vi "Publish and Subscribe Event-based.vi"() -> ()   [LabVIEW 2020]
uses:
  <userlib>/lvwamp/WAMP Client/WAMP Client.lvclass/WAMP Client.ctl
  <userlib>/lvwamp/WAMP Client/Accessors/Read Daemon Stopped.vi
  <userlib>/lvwamp/WAMP Client/New WebSocket Client.vi
  <userlib>/lvwamp/WAMP Client/WAMP Client.lvclass
panel:
  out "Error URI":string
  out "Callee Error?":bool
  out "Call Result ArgumentKw":string
  out "Call Result Arguments":string[](array[string])
  in  "Call Arguments":string[](array[string])
  in  "Call URI":string="test.topic"
  in  "Call":bool caption="Publish Topic"
  in  "Unsubscribe":bool caption="Publish Topic"
  out "Topic:":string
  out "ArgumentKw Payload":string
  out "Arguments Payload":string[](array[string])
  out "Event received on:":string
  in  "Publish Argument Payload":string[](array[string])
  in  "Subscription URI":string="test.topic"
  in  "Subscribe":bool caption="Publish Topic"
  in  "Disconnect":bool caption="Publish Topic"
  in  "Realm":string="default_realm"
  in  "Topic URI":string="test.topic"
  in  "Publish":bool caption="Publish Topic"
  in  "Port":u16=55555
  in  "Router Address":string="localhost"
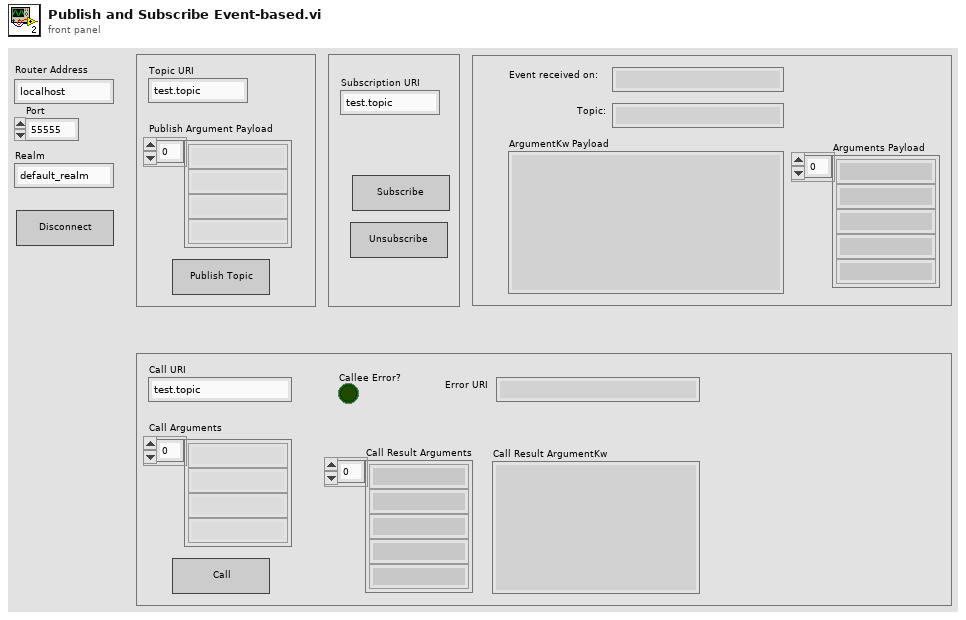
[diagram p1: front panel]
types:
  T1 = typedef "WAMP Client.lvclass/WAMP Error Payload.ctl" = cluster{"Arguments Payload":string[], "ArgumentKw Payload":string, "Error URI":string, "Error?":bool}
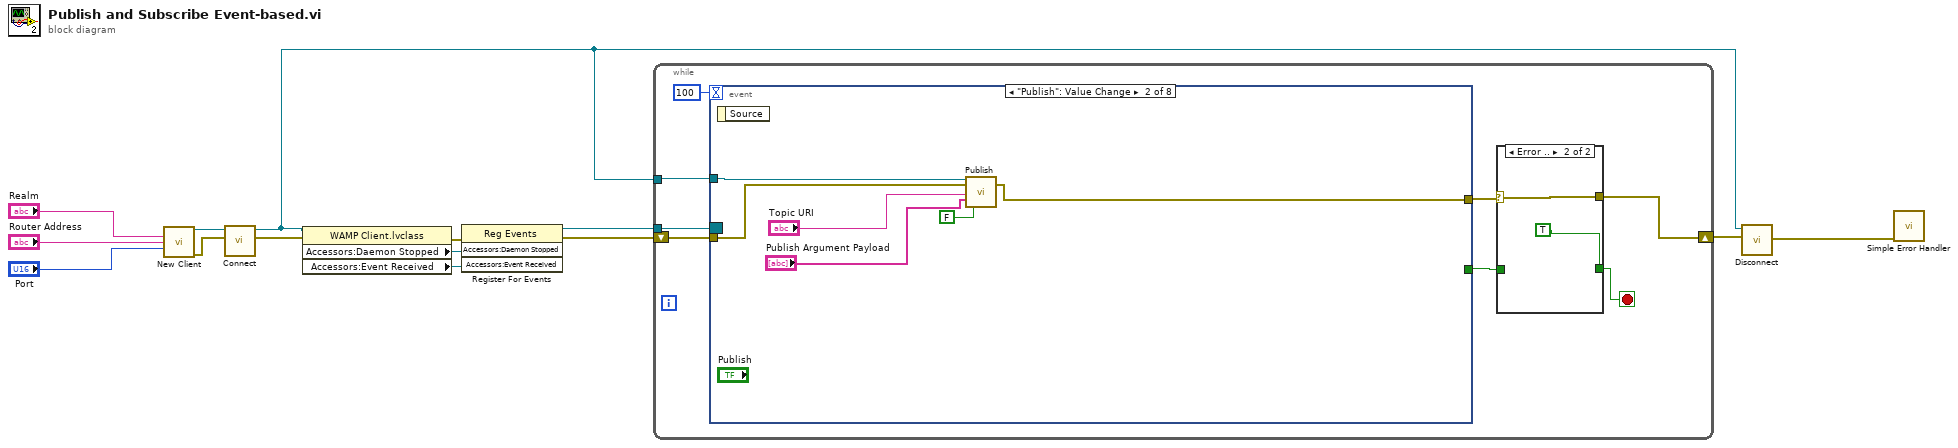
[diagram p0: block diagram]
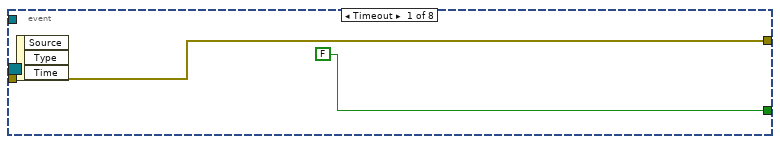
[diagram p3: hidden frame]
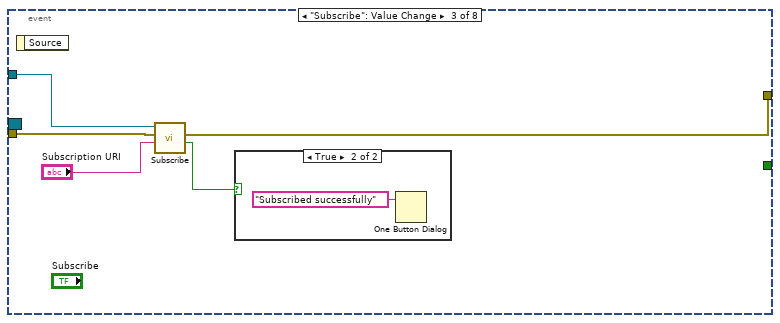
[diagram p4: hidden frame]
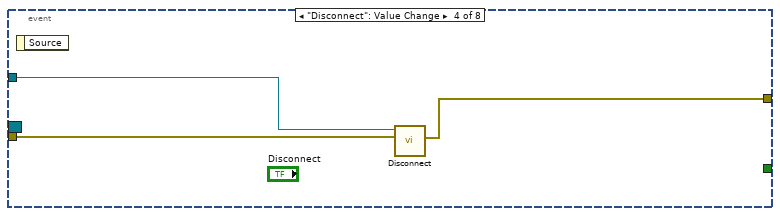
[diagram p6: hidden frame]
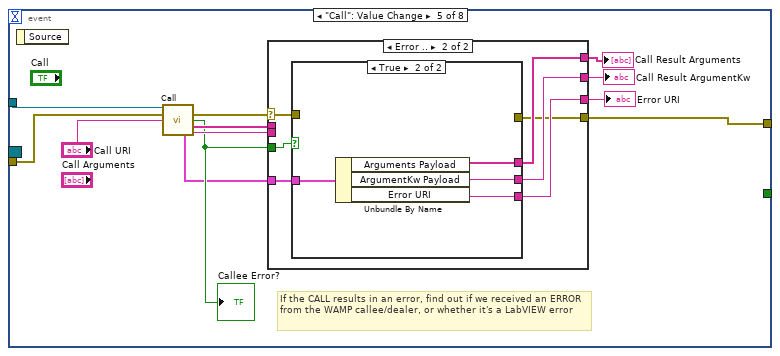
[diagram p7: hidden frame]
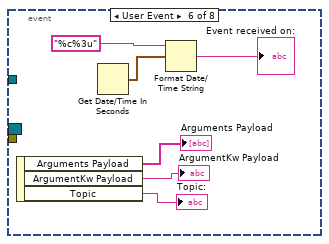
[diagram p10: hidden frame]
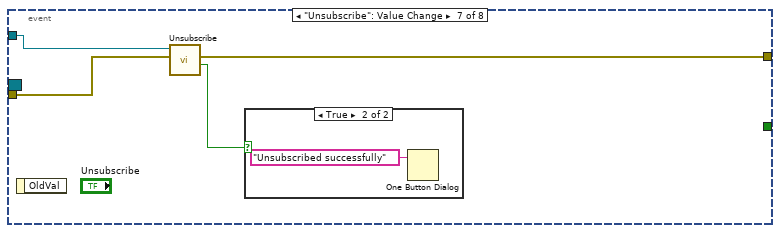
[diagram p11: hidden frame]
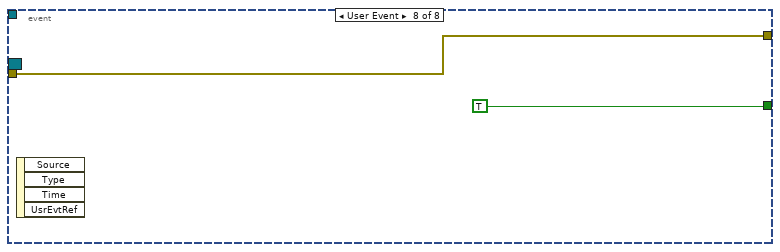
[diagram p13: hidden frame]
diagram:
  n1 = call-poly <userlib>:"New Client.vi"("Realm"="Realm", "Address"="Router Address", "Port"="Port") -> ("reference out"=w11:refnum<class "WAMP Client.lvclass">, "error out"=w8:errorcluster)  [unwired: 11 in]
  n2 = call <userlib>:"Connect.vi"("error in (no error)"=w8, "WAMP Client in"=w11) -> ("error out"=w2:errorcluster, "WAMP Client out"=w3:refnum<class "WAMP Client.lvclass">)  [unwired: 8 in]
  n3 = property class="WAMP Client.lvclass"(reference=w3, error in=w2) -> (error out=w9:errorcluster, "Accessors:Daemon Stopped"=w10:refnum<user-event>, "Accessors:Event Received"=w5:refnum<user-event>)  [unwired: 1 out]
  n4 = register-events(error in=w9, w10, w5) -> (reference out=w6:refnum<event-registration>, error out=w4:errorcluster)  [unwired: 1 in]
  n5 = while {
    tunnel: w3 -> [w22]
    shift-right: [w20] -> w7
    shift-left: w4 -> [w18]
    tunnel: w6 -> [w19]
    stop <- w16 stop-if-true
    n6 = event shown="[1] \"Publish\": Value Change" {
      selector: w19 -> [_ _ _ _ _ _ _ _]
      dyn-events: _ -> [_ _ _ _ _ _ _ _]
      timeout: 100 -> [_ _ _ _ _ _ _ _]
      tunnel: w22 -> [_ w34 w39 w43 w55 _ w79 _]
      tunnel: [FALSE _ _ _ _ _ _ TRUE] -> w17
      tunnel: w18 -> [w27 w33 w38 w41 w54 _ w80 w82]
      tunnel: [w27 w32 w37 w42 w51 _ w78 w82] -> w21
      event Timeout {
        n7 = event-data() -> ()  [unwired: 1 in, 3 out]
      }
      event "Publish": Value Change {
        n8 = event-data() -> ()  [unwired: 1 in, 1 out]
        n9 = call-dynamic "Publish.vi"("WAMP Client in"=w34, "error in (no error)"=w33, "Topic"="Topic URI", "Arguments"="Publish Argument Payload", "Request Ack."=FALSE) -> ("error out"=w32:errorcluster)  [unwired: 13 in, 1 out]
      }
      event "Subscribe": Value Change {
        n10 = event-data() -> ()  [unwired: 1 in, 1 out]
        n11 = call-dynamic "Subscribe.vi"("Topic"="Subscription URI", "error in (no error)"=w38, "WAMP Client in"=w39) -> ("Success?"=w36:bool, "error out"=w37:errorcluster)  [unwired: 3 in, 2 out]
        n12 = case shown="True" w36 {
          frame False {
          }
          frame True {
            n13 = One Button Dialog(message="Subscribed successfully") -> ()  [unwired: 1 in, 1 out]
          }
        }
      }
      event "Disconnect": Value Change {
        n14 = event-data() -> ()  [unwired: 1 in, 1 out]
        n15 = call-dynamic "Disconnect.vi"("error in (no error)"=w41, "WAMP Client in"=w43) -> ("error out"=w42:errorcluster)  [unwired: 8 in, 1 out]
      }
      event "Call": Value Change {
        # "If the CALL results in an error, find out if we received an ERROR from the WAMP callee/dealer, or whether it's a LabVIEW error"
        n16 = event-data() -> ()  [unwired: 1 in, 1 out]
        n17 = call-dynamic "Call.vi"("WAMP Client in"=w55, "error in (no error)"=w54, "Topic URI"="Call URI") -> ("error out"=w52:errorcluster, "Callee Error?"=w46:bool, "Arguments Payload"=w49:string[], "WAMP Error"=w44:T1, "ArgumentKw Payload"=w48:string)  [unwired: 7 in, 1 out]
        "Callee Error?" <- w46
        n18 = case shown="Error .." w52 {
          selector: w52 -> [w58 w60]
          tunnel: [w58 w59] -> w51
          tunnel: [w57 w63] -> w50
          tunnel: w49 -> [w57 _]
          tunnel: w48 -> [w56 _]
          tunnel: [w56 w62] -> w47
          tunnel: w46 -> [_ w65]
          tunnel: [_ w61] -> w45
          tunnel: w44 -> [_ w64]
          frame No Error {
          }
          frame Error {
            n19 = case shown="True" w65 {
              tunnel: w64 -> [_ w70]
              tunnel: [_ w69] -> w63
              tunnel: [_ w68] -> w62
              tunnel: [_ w67] -> w61
              tunnel: w60 -> [w66 _]
              tunnel: [w66 _] -> w59
              frame False {
              }
              frame True {
                n20 = Unbundle By Name(w70) -> ("Arguments Payload"=w69:string[], "ArgumentKw Payload"=w68:string, "Error URI"=w67:string)
              }
            }
          }
        }
        "Call Result Arguments" <- w50
        "Call Result ArgumentKw" <- w47
        "Error URI" <- w45
      }
      event User Event {
        n21 = event-data() -> ("Arguments Payload"=→"Arguments Payload":string[], "ArgumentKw Payload"=→"ArgumentKw Payload":string, "Topic"=→"Topic:":string)  [unwired: 1 in]
        n22 = Get Date/Time In Seconds() -> (seconds since 1Jan1904=w76:timestamp)
        n23 = Format Date/Time String(time format string (%c)="%c%3u", seconds (now)=w76) -> (date/time string=→"Event received on:":string)  [unwired: 1 in]
      }
      event "Unsubscribe": Value Change {
        n24 = event-data() -> ()  [unwired: 1 in, 1 out]
        n25 = call-dynamic "Unsubscribe.vi"("error in (no error)"=w80, "WAMP Client in"=w79) -> ("Success?"=w77:bool, "error out"=w78:errorcluster)  [unwired: 5 in, 1 out]
        n26 = case shown="True" w77 {
          frame False {
          }
          frame True {
            n27 = One Button Dialog(message="Unsubscribed successfully") -> ()  [unwired: 1 in, 1 out]
          }
        }
      }
      event User Event {
        n28 = event-data() -> ()  [unwired: 1 in, 4 out]
      }
    }
    n29 = case shown="Error .." w21 {
      selector: w21 -> [w24 w25]
      tunnel: [w23 TRUE] -> w16
      tunnel: [w24 w25] -> w20
      tunnel: w17 -> [w23 _]
      frame No Error {
      }
      frame Error {
      }
    }
  }
  n30 = call-dynamic "Disconnect.vi"("error in (no error)"=w7, "WAMP Client in"=w3) -> ("error out"=w1:errorcluster)  [unwired: 8 in, 1 out]
  n31 = call <vilib>:"Simple Error Handler.vi"("error in (no error)"=w1) -> ()  [unwired: 4 in, 5 out]
